vi "SCALE_MOVE.vi"(6 "ARM 2 FEEDBACK":dbl, 7 "RESET":bool, 8 "ARM 1 FEEDBACK":dbl, 9 "ARM 2 INITIAL":dbl, 10 "ARM 1 INITIAL":dbl, 11 "INPUT":bool) -> (0 "ARM 2 SETPOINT OUT":dbl, 2 "RUNNING?":bool, 3 "ARM 1 SETPOINT OUT":dbl)   [LabVIEW 2017]
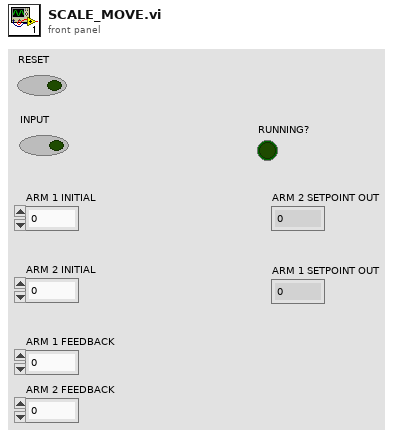
[diagram p1: front panel]
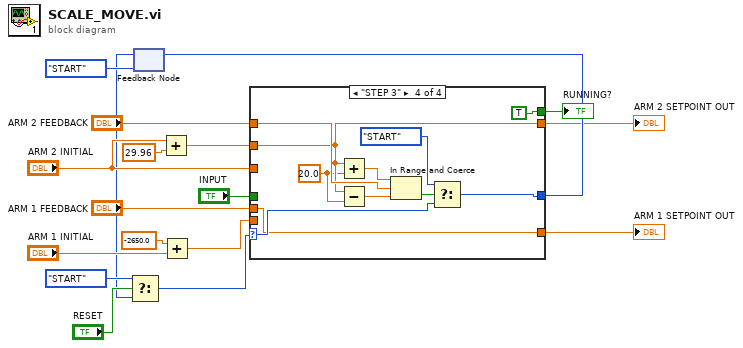
[diagram p0: block diagram]
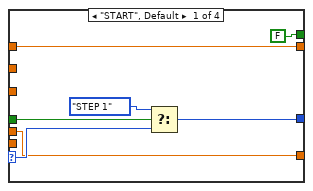
[diagram p2: hidden frame]
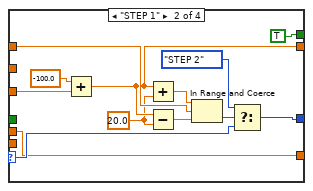
[diagram p3: hidden frame]
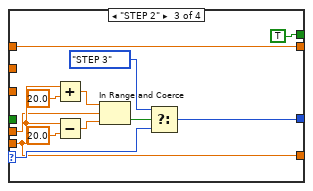
[diagram p4: hidden frame]
diagram:
  n1 = feedback #1(enum16{"START", "STEP 1", "STEP 2", "STEP 3"}."START") -> (w2:enum16{"START", "STEP 1", "STEP 2", "STEP 3"})
  n2 = Select(t=enum16{"START", "STEP 1", "STEP 2", "STEP 3"}."START", s="RESET", f=w2) -> (s? t:f=w1:enum16{"START", "STEP 1", "STEP 2", "STEP 3"})
  n3 = Add(x="ARM 2 INITIAL", y=29.96) -> (x+y=w8:dbl)
  n4 = Add(x=-2650.0, y="ARM 1 INITIAL") -> (x+y=w6:dbl)
  n5 = case shown="\"STEP 3\"" w1 {
    selector: w1 -> [w24 w38 w50 w61]
    tunnel: [w25 w37 w49 w60] -> w17
    tunnel: "INPUT" -> [w23 _ _ _]
    tunnel: w6 -> [_ _ w41 _]
    tunnel: w8 -> [_ _ _ w52]
    tunnel: "ARM 2 FEEDBACK" -> [w20 w32 w39 w55]
    tunnel: [w20 w27 w39 w52] -> w14
    tunnel: "ARM 1 FEEDBACK" -> [w21 w34 w40 w58]
    tunnel: [w21 w34 w41 w58] -> w12
    tunnel: [FALSE TRUE TRUE TRUE] -> w11
    tunnel: "ARM 2 INITIAL" -> [_ w31 _ _]
    frame "START", Default {
      n6 = Select(t=enum16{"START", "STEP 1", "STEP 2", "STEP 3"}."STEP 1", s=w23, f=w24) -> (s? t:f=w25:enum16{"START", "STEP 1", "STEP 2", "STEP 3"})
    }
    frame "STEP 1" {
      w26 = 20.0 ("y")
      n7 = Add(x=-100.0, y=w31) -> (x+y=w27:dbl)
      n8 = Add(x=w27, y=w26) -> (x+y=w28:dbl)
      n9 = Subtract(x=w27, y=w26) -> (x-y=w29:dbl)
      n10 = In Range and Coerce(upper limit=w28, x=w32, lower limit=w29) -> (In Range?=w33:bool)  [unwired: 1 out]
      n11 = Select(t=enum16{"START", "STEP 1", "STEP 2", "STEP 3"}."STEP 2", s=w33, f=w38) -> (s? t:f=w37:enum16{"START", "STEP 1", "STEP 2", "STEP 3"})
    }
    frame "STEP 2" {
      n12 = Add(x=w41, y=20.0) -> (x+y=w45:dbl)
      n13 = Subtract(x=w41, y=20.0) -> (x-y=w44:dbl)
      n14 = In Range and Coerce(upper limit=w45, x=w40, lower limit=w44) -> (In Range?=w46:bool)  [unwired: 1 out]
      n15 = Select(t=enum16{"START", "STEP 1", "STEP 2", "STEP 3"}."STEP 3", s=w46, f=w50) -> (s? t:f=w49:enum16{"START", "STEP 1", "STEP 2", "STEP 3"})
    }
    frame "STEP 3" {
      w51 = 20.0 ("y")
      n16 = Add(x=w52, y=w51) -> (x+y=w53:dbl)
      n17 = Subtract(x=w52, y=w51) -> (x-y=w54:dbl)
      n18 = In Range and Coerce(upper limit=w53, x=w55, lower limit=w54) -> (In Range?=w56:bool)  [unwired: 1 out]
      n19 = Select(t=enum16{"START", "STEP 1", "STEP 2", "STEP 3"}."START", s=w56, f=w61) -> (s? t:f=w60:enum16{"START", "STEP 1", "STEP 2", "STEP 3"})
    }
  }
  "ARM 2 SETPOINT OUT" <- w14
  "ARM 1 SETPOINT OUT" <- w12
  "RUNNING?" <- w11
  n20 = feedback-in #1(w17) -> ()
